vi "templates table BODY data keys.vi"(9 "Template Keys":T1, 10 "HTM Keys":T1) -> (2 "HTM Keys":T1)   [LabVIEW 2011]
uses:
  ITK EXT/utils/keyedarr.llb/Keyed Array.ctl
  ITK EXT/utils/strutil.llb/Case Matching.ctl
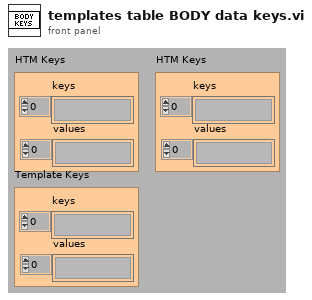
[diagram p1: front panel]
types:
  T1 = typedef "Keyed Array.ctl" = cluster{"keys":string[], "values":string[]}
  T2 = typedef "Case Matching.ctl" = enum16{"a != A", "a == A", "system"}
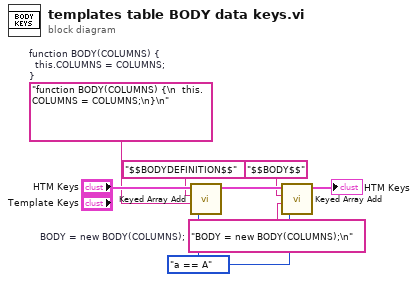
[diagram p0: block diagram]
diagram:
  w2 = "BODY = new BODY(COLUMNS);\n"  # BODY = new BODY(COLUMNS);
  w1 = Case_Matching."a == A" ("case matching (sensitive)")
  w6 = "function BODY(COLUMNS) {\n  this.COLUMNS = COLUMNS;\n}\n"  # function BODY(COLUMNS) {   this.COLUMNS = COLUMNS; }
  n1 = call "Keyed Array Add.vi"("case matching (sensitive)"=w1, "value"=w6, "key"="$$BODYDEFINITION$$", "array in"="HTM Keys") -> ("array out"=w5:T1)  [unwired: 3 out]
  n2 = call "Keyed Array Add.vi"("case matching (sensitive)"=w1, "value"=w2, "key"="$$BODY$$", "array in"=w5) -> ("array out"=→"HTM Keys":T1)  [unwired: 3 out]
